vi "make_stim_digital_protocol.vi"(8 "Error in":errorcluster, 10 "Device parameters":T1={"Triggered?"=FALSE, "Shutter channel"="", "Acquisition channels"="", "Acquisition sample rate"=1000.0, "Read chunk size"=100, "Stimulation channel"="Dev1/ao0", "Stimulation sample rate"=100.0} {"Read chunk size" min=100 max=100000; "Acquisition sample rate" min=10.0 max=10000.0 step=10.0; "Stimulation sample rate" min=10.0 max=10000.0}, 11 "Protocol parameters":T2={"Repetitions"=1.0, "ON time"=40.0, "OFF time"=120.0, "Stim onset"=5.0, "Stim frequency"=1.0, "Pulse width"=1.0, "Acquire before ON"=1.0, "Acquire after ON"=1.0, "Sync shutter to acquisition"=TRUE} {"Pulse width" min=0.0001 max=0.1 step=0.01; "Acquire after ON" min=0.0 max=10.0 step=1.0; "Acquire before ON" min=0.0 max=10.0 step=1.0; "Repetitions" min=1.0 max=10.0 step=1.0; "OFF time" min=0.0 max=1000.0; "ON time" min=0.0 max=1000.0; "Stim onset" min=0.0 max=100.0; "Stim frequency" min=0.1 max=40.0 step=1.0}) -> (0 "Error out":errorcluster, 2 "Stim digital array":u8[](array[numeric]))   [LabVIEW 2010]
uses:
  typedefs/protocol_parameters.ctl
  typedefs/device_parameters.ctl
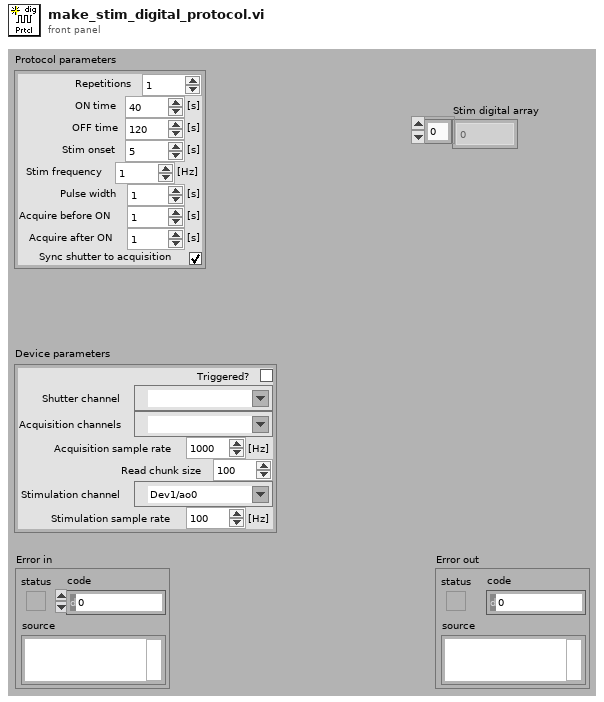
[diagram p1: front panel]
types:
  T1 = typedef "device_parameters.ctl" = cluster{"Triggered?":bool, "Shutter channel":tag, "Acquisition channels":tag, "Acquisition sample rate":dbl, "Read chunk size":i32, "Stimulation channel":tag, "Stimulation sample rate":dbl}
  T2 = typedef "protocol_parameters.ctl" = cluster{"Repetitions":dbl, "ON time":dbl, "OFF time":dbl, "Stim onset":dbl, "Stim frequency":dbl, "Pulse width":dbl, "Acquire before ON":dbl, "Acquire after ON":dbl, "Sync shutter to acquisition":bool}
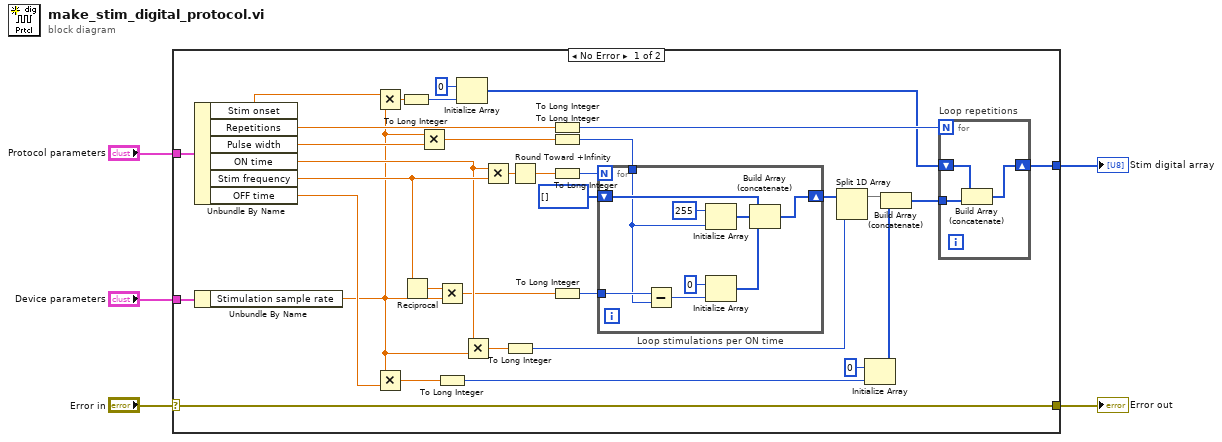
[diagram p0: block diagram]
diagram:
  n1 = case shown="No Error" "Error in" {
    selector: "Error in" -> [w37 w52]
    tunnel: [w37 w52] -> w4
    tunnel: "Protocol parameters" -> [w39 _]
    tunnel: "Device parameters" -> [w31 _]
    tunnel: [w16 _] -> w1
    frame No Error {
      n2 = Unbundle By Name(w39) -> ("Stim onset"=w15:dbl, "Repetitions"=w14:dbl, "Pulse width"=w13:dbl, "ON time"=w32:dbl, "Stim frequency"=w34:dbl, "OFF time"=w33:dbl)
      n3 = Unbundle By Name(w31) -> ("Stimulation sample rate"=w12:dbl)
      n4 = Multiply(x=w15, y=w12) -> (x*y=w11:dbl)
      n5 = Multiply(x=w12, y=w33) -> (x*y=w21:dbl)
      n6 = To Long Integer(number=w11) -> (32bit integer=w10:i32)
      n7 = Reciprocal(x=w34) -> (1/x=w30:dbl)
      n8 = Multiply(x=w12, y=w13) -> (x*y=w7:dbl)
      n9 = Multiply(x=w30, y=w12) -> (x*y=w9:dbl)
      n10 = To Long Integer(number=w21) -> (32bit integer=w20:i32)
      n11 = Initialize Array(u8 0 ("element"), w10) -> (w17:u8[])
      n12 = Multiply(x=w32, y=w12) -> (x*y=w29:dbl)
      n13 = Multiply(x=w32, y=w34) -> (x*y=w36:dbl)
      n14 = To Long Integer(number=w29) -> (32bit integer=w24:i32)
      n15 = Round Toward +Infinity(x=w36) -> (ceil(x): smallest int >= x=w35:dbl)
      n16 = To Long Integer(number=w14) -> (32bit integer=w19:i32)
      n17 = To Long Integer(number=w7) -> (32bit integer=w6:i32)
      n18 = To Long Integer(number=w35) -> (32bit integer=w26:i32)
      n19 = To Long Integer(number=w9) -> (32bit integer=w8:i32)
      n20 = for "Loop stimulations per ON time" {
        N: w26 -> [_]
        tunnel: w8 -> [w50]
        tunnel: w6 -> [w44]
        shift-right: [w45] -> w25
        shift-left: u8[] [] -> [w46]
        n21 = Subtract(x=w50, y=w44) -> (x-y=w43:i32)
        n22 = Initialize Array(u8 255 ("element"), w44) -> (w48:u8[])
        n23 = Initialize Array(u8 0 ("element"), w43) -> (w47:u8[])
        n24 = Build Array (concatenate)(w46, w48, w47) -> (w45:u8[])
      }
      n25 = Split 1D Array(array=w25, index=w24) -> (first subarray=w22:u8[])  [unwired: 1 out]
      n26 = Initialize Array(u8 0 ("element"), w20) -> (w27:u8[])
      n27 = Build Array (concatenate)(w22, w27) -> (w18:u8[])
      n28 = for "Loop repetitions" {
        N: w19 -> [_]
        shift-right: [w40] -> w16
        shift-left: w17 -> [w42]
        tunnel: w18 -> [w41]
        n29 = Build Array (concatenate)(w42, w41) -> (w40:u8[])
      }
    }
    frame Error {
    }
  }
  "Error out" <- w4
  "Stim digital array" <- w1
